vi "SAC-Add Filestem to Ring.vi"(0 "Ring in":refnum<vi>, 7 "filename":string) -> ()   [LabVIEW 2020]
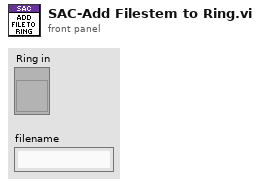
[diagram p1: front panel]
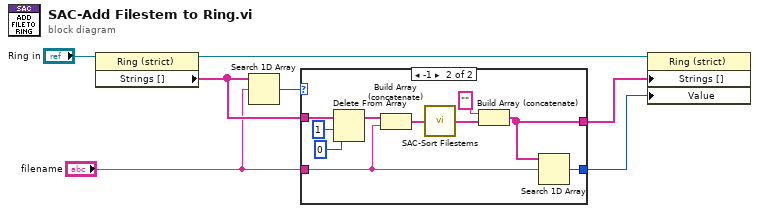
[diagram p0: block diagram]
diagram:
  n1 = property on="Property Node" class="Ring (strict)"(reference="Ring in") -> (reference out=w6:refnum<vi>, "Strings []"=w4:string[])  [unwired: 1 in, 1 out]
  n2 = Search 1D Array(1D array=w4, element="filename") -> (index of element=w5:i32)  [unwired: 1 in]
  n3 = case shown="-1" w5 {
    selector: w5 -> [w8 _]
    tunnel: [w9 w11] -> w3
    tunnel: "filename" -> [_ w18]
    tunnel: w4 -> [w9 w19]
    tunnel: [w8 w17] -> w1
    frame 0, Default {
    }
    frame -1 {
      n4 = Delete From Array(array=w19, length=1, index=0) -> (array with subset deleted=w14:string[])  [unwired: 1 out]
      n5 = Build Array (concatenate)(w14, w18) -> (w16:string[])
      n6 = call "SAC-Sort Filestems.vi"("Filestems"=w16) -> ("Sorted filestems"=w15:string[])  [unwired: 14 in]
      n7 = Build Array (concatenate)("", w15) -> (w11:string[])
      n8 = Search 1D Array(1D array=w11, element=w18) -> (index of element=w17:i32)  [unwired: 1 in]
    }
  }
  n9 = property on="Property Node" class="Ring (strict)"(reference=w6, "Strings []"=w3, "Value"=w1) -> ()  [unwired: 1 in, 2 out]
